vi "1_Installation.vi"() -> ()   [LabVIEW 2026]
panel:
  out "Sine":dynamicdata(graph)
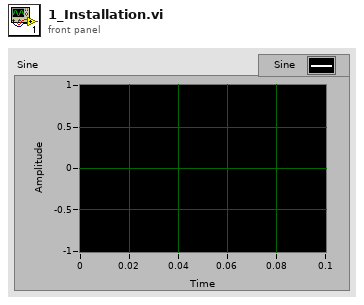
[diagram p1: front panel]
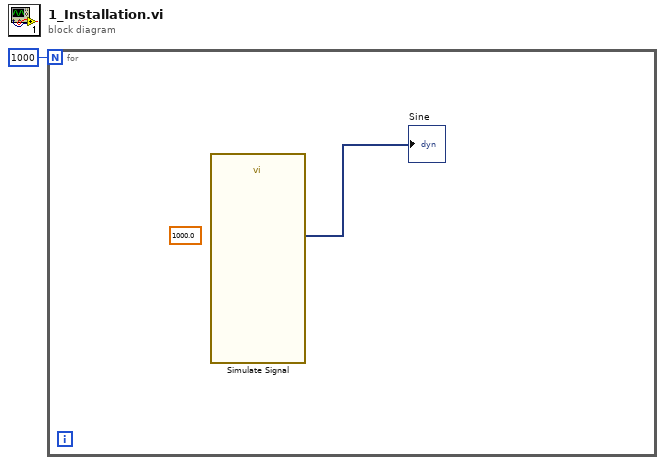
[diagram p0: block diagram]
diagram:
  n1 = for {
    N: 1000 -> [_]
    (unwired) 1000.0 ("Sine")
    n2 = call "Simulate Signal"() -> ("Sine"=→"Sine":dynamicdata)  [unwired: 14 in, 1 out]
  }
